vi "Calibration Process.vi"(5 "Sum in":dbl, 6 "DONE?":bool, 7 "CONFIG CALIBRATION":T1, 8 "error in":errorcluster, 9 "Index":i32, 10 "Current Valve":dbl, 11 "Queue in":refnum<queue>) -> (0 "error out":errorcluster, 3 "Sum out":dbl)   [LabVIEW 2018]
uses:
  Controls/ConfigCalibration.ctl
  Message Queue/Message Cluster.ctl
  Message Queue/Message.ctl
  Controls/Calibration Cluster.ctl
  Message Queue/Message Queue.lvlib
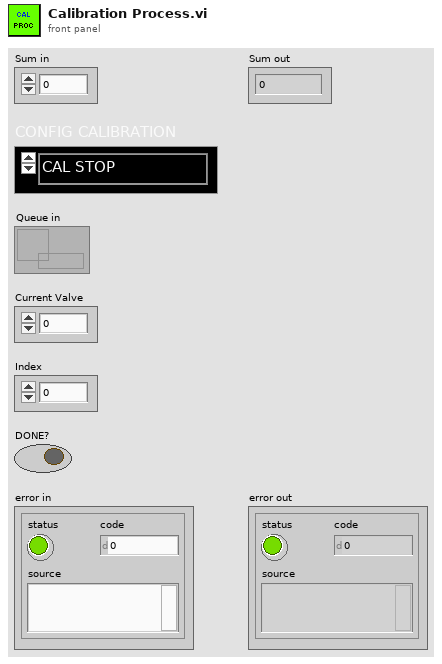
[diagram p1: front panel]
types:
  T1 = typedef "ConfigCalibration.ctl" = enum16{"CAL STOP", "TWTT OP (IN)", "TWTT PDP (IN)", "DLT OP (IN)", "DLT PDP 01 (IN)", "DLT PDP 02 (IN)", "BR OP (IN)", "BR TWT ALIGN (IN)", "BR DL ALIGN (IN)"}
  T2 = typedef "Calibration Cluster.ctl" = cluster{"CONFIG CALIBRATION":T1, "Calibration Value":dbl}
  T3 = typedef "Message Queue.lvlib/Message.ctl" = enum16{"Initialize", "Initialize UI Refs", "Disable Controls", "Enable UI Controls", "Connect RT", "Get Control Mode from RT", "Send Control Mode to UI", "Update Control Mode", "Get Config from RT", "Send Config to UI", "Update Parameters", "Change Parameters", "Calibrate Config", "Update Calibration", "Change Valve State", "Get Valve Status from RT", "Send Valve Status to UI", "Update Valve Status", "Inital UI Values", "Disconnect RT", "Close Connection", "Disconnect UI", "Run Mode", "Stop ALL", "Change Control Mode", "Skid Manual", "Computer Manual", "Step Automated", "Fully Automated", "Reset", "Pumps Command", "Pump State Changed", "Critical Error", "Log-Only Error", "Non-Critical Error", "RT Error", "Update System Status", "Update DI Status", "Clear System Status", "Update Warning", "Clear Warning", "Upate Timeout", "Update Reset Status", "Waiting", "Verify Password", "Manual Cleaning Process", "Update Manual Cleaning Process", "Cal - Body", "Cal - US", "Cal - Update Parameters", "Propotional Update", "Exit", "---Copy This Frame---"}
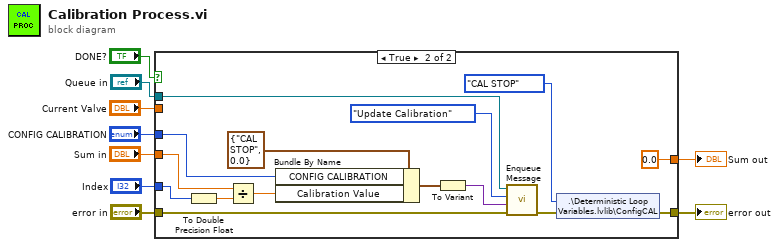
[diagram p0: block diagram]
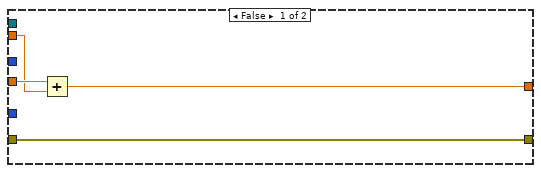
[diagram p2: hidden frame]
diagram:
  n1 = case shown="True" "DONE?" {
    tunnel: "Sum in" -> [w12 w25]
    tunnel: "Current Valve" -> [w11 _]
    tunnel: [w10 0.0] -> w6
    tunnel: "error in" -> [w13 w20]
    tunnel: [w13 w28] -> w5
    tunnel: "Index" -> [_ w19]
    tunnel: "Queue in" -> [_ w22]
    tunnel: "CONFIG CALIBRATION" -> [_ w16]
    frame False {
      n2 = Add(x=w12, y=w11) -> (x+y=w10:dbl)
    }
    frame True {
      n3 = To Double Precision Float(number=w19) -> (double precision float=w18:dbl)
      n4 = Divide(x=w25, y=w18) -> (x/y=w15:dbl)
      n5 = Bundle By Name(cluster=T2 {"CONFIG CALIBRATION"=enum."CAL STOP", "Calibration Value"=0.0} ("Calibration Cluster"), "CONFIG CALIBRATION"=w16, "Calibration Value"=w15) -> (w14:T2)
      n6 = To Variant(anything=w14) -> (Variant=w23:variant)
      n7 = call "Enqueue Message.vi"("error in (no error)"=w20, "Message Data"=w23, "Message"=Message."Update Calibration", "Message Queue"=w22) -> ("error out"=w24:errorcluster)  [unwired: 6 in, 1 out]
      n8 = shared-variable ".\\Deterministic Loop Variables.lvlib\\ConfigCAL"(ConfigCalibration."CAL STOP" ("ConfigCAL"), error in=w24) -> (error out=w28:errorcluster)
    }
  }
  "Sum out" <- w6
  "error out" <- w5
